vi "Measure Single.vi"(8 "error in (no error)":errorcluster, 11 "DMM Driver in":refnum<class "DMM Driver.lvclass">) -> (0 "error out":errorcluster, 1 "Config":T1={"Function"=enum."DC Volts", "Range"=0.0, "Digit Resolution(5½)"=enum."5½"}, 2 "Measurement":dbl=nan, 3 "DMM Driver out":refnum<class "DMM Driver.lvclass">, 4 "Valid measurement?":bool, 5 "Finished?":bool)   [LabVIEW 2020, in "DMM.lvlib" / "DMM Driver.lvclass"]
doc: "Perform a single measurement on the DMM if time allows and return the measurement and current DMM configuration."
uses:
  DMM Driver.lvclass
  Controls/Ctl_DigitResolution.ctl
  DMM.lvlib
  Controls/Ctl_Function.ctl
  Controls/Community/Ctl_Config.ctl
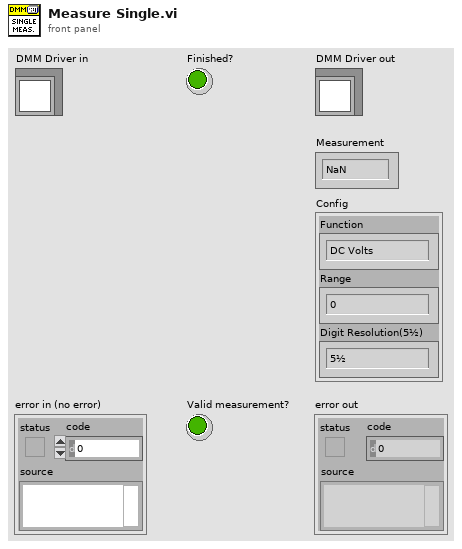
[diagram p1: front panel]
types:
  T1 = typedef "DMM.lvlib/Ctl_Config.ctl" = cluster{"Function":T2, "Range":dbl, "Digit Resolution(5½)":T3}
  T2 = typedef "DMM.lvlib/Ctl_Function.ctl" = enum8{"DC Volts", "AC Volts", "DC Current", "AC Current", "2-wire Resistance", "4-wire Resistance", "Diode", "Frequency", "Period", "AC Volts DC Coupled", "Capacitance", "Inductance", "Temperature"}
  T3 = typedef "DMM.lvlib/Ctl_DigitResolution.ctl" = enum8{"3½", "4½", "5½", "6½", "7½"}
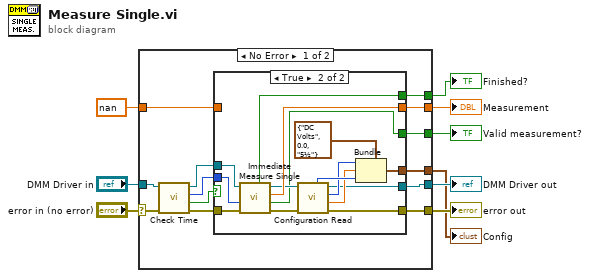
[diagram p0: block diagram]
diagram:
  n1 = case shown="No Error" "error in (no error)" {
    selector: "error in (no error)" -> [w20 w43]
    tunnel: [w17 w43] -> w8
    tunnel: [w19 w42] -> w6
    tunnel: "DMM Driver in" -> [w22 w42]
    tunnel: [w14 w41] -> w5
    tunnel: [w13 _] -> w4
    tunnel: [w12 _] -> w3
    tunnel: [w11 _] -> w2
    tunnel: nan ("Measurement") -> [w10 w41]
    frame No Error {
      n2 = call "Check Time.vi"("error in (no error)"=w20, "DMM Driver in"=w22) -> ("error out"=w16:errorcluster, "Time OK?"=w21:bool, "Remaining Time"=w15:i32, "DMM Driver out"=w18:refnum<class "DMM Driver.lvclass">)  [unwired: 6 in]
      n3 = case shown="True" w21 {
        tunnel: [w25 w31] -> w19
        tunnel: w18 -> [w25 w40]
        tunnel: [w24 w29] -> w17
        tunnel: w16 -> [w24 w38]
        tunnel: w15 -> [_ w39]
        tunnel: [w23 w37] -> w14
        tunnel: [_ w28] -> w13
        tunnel: [_ w27] -> w12
        tunnel: [_ w26] -> w11
        tunnel: w10 -> [w23 _]
        frame False {
        }
        frame True {
          n4 = call-dynamic "Immediate Measure Single.vi"("error in (no error)"=w38, "Max Time (-1ms)"=w39, "DMM Driver in"=w40) -> ("error out"=w30:errorcluster, "Valid measurement?"=w26:bool, "Measurement"=w37:dbl, "DMM Driver out"=w32:refnum<class "DMM Driver.lvclass">, "Finished?"=w27:bool)  [unwired: 4 in]
          n5 = call-dynamic "Configuration Read.vi"("error in (no error)"=w30, "DMM Driver in"=w32) -> ("error out"=w29:errorcluster, "Range"=w35:dbl, "Function"=w34:T2, "DMM Driver out"=w31:refnum<class "DMM Driver.lvclass">, "Digit Resolution(5½)"=w36:T3)  [unwired: 5 in]
          n6 = Bundle(cluster=T1 {"Function"=enum."DC Volts", "Range"=0.0, "Digit Resolution(5½)"=enum."5½"} ("Config"), "Function"=w34, "Range"=w35, "Digit Resolution(5½)"=w36) -> (w28:T1)
        }
      }
    }
    frame Error {
    }
  }
  "error out" <- w8
  "DMM Driver out" <- w6
  "Config" <- w4
  "Measurement" <- w5
  "Valid measurement?" <- w2
  "Finished?" <- w3
